vi "mainVI.vi"() -> ()   [LabVIEW 2019]
uses:
  controls/#typedef_StateMachine_States.ctl
  <vilib>/sound2/lvsound2.llb/Sampling Mode.ctl
  controls/#typedef_Waveform_Type.ctl
  <vilib>/sound2/lvsound2.llb/Sound Data Format.ctl
  <vilib>/sound2/lvsound2.llb/Sound Output Task ID.ctl
  controls/#typedef_Data_Cluster.ctl
  <vilib>/Utility/file.llb/Read Delimited Spreadsheet (string).vi
  <vilib>/sound2/lvsound2.llb/Sound Output Write (DBL Single).vi
panel:
  out "Main Data Cluster":T1={"Notes Frequency Array"=[], "Main Waveform Type"=enum."Sine", "Waveform"={"t0"=timestamp(0 s since 1904-01-01), "dt"=1.0, "Y"=[]}, "Main Current Note"=0, "Octave Range Offset"=0, "sound format"={"sample rate (S/s)"=22050.0, "number of channels"=2, "bits per sample"=16}, "Task ID"=0, "Note Duration"=0.0, "Volume"=0.0, "ADSR Envelope Cluster"={"Decay"=0, "Sustain"=0, "Attack"=0, "Release"=0}, "Playing?"=FALSE, "Pitch LFO"={"Rate"=0.0, "Ammount"=0.0}, "device ID"=0, "Filter Section"={"Lowpass Freq"=0.0, "Highpass Freq"=0.0, "Enable"=FALSE}, "Distortion"={"Distortion level"=0.0, "Enable"=FALSE}, "Secondary Waveform Type"=enum."Sine", "Secondary Frequency"=0.0, "Secondary Blend"=0.0, "Envelope XY Graph"={[], []}, "Buffer Number"=0, "End of Sequence?"=FALSE} {"task ID" format="%.0x"}
  out "error out":errorcluster
  out "ADSR Graph":cluster{dbl[], dbl[]}(graph)
  in  "Load Button":bool
  in  "Save Button":bool
  in  "Filter frequency":dbl(slide)=5.783132530120482 min=-0.0 max=1125.0 scale=1.0..1125.0 scale format="%#_5g"
  out "Waveform Graph":waveform(dbl)(graph)
  in  "Octave Range":u32(knob)=2 min=1 max=4 step=1 scale=1.0..4.0
  in  "Sub Volume":dbl(knob) scale=0.0..1.0
  in  "Sub Waveform Selection":u32(knob) max=4 step=1 scale=0.0..4.0
  in  "Sub Note Dial":dbl(knob) min=0.0 step=1.0 scale=0.0..12.0
  in  "Distortion level":dbl(slide) scale=0.0..100.0
  out "Distortion Enable LED":bool
  in  "Distortion Enable":bool
  out "Filter Enable LED":bool
  in  "Filter Enable":bool
  in  "Waveform Selection":u32(knob) max=4 step=1 scale=0.0..4.0
  in  "Pause Button":bool
  in  "Play Button":bool
  in  "Stop Button":bool
  in  "Volume":dbl(knob) scale=0.0..1.0
  in  "Sustain":i32(slide)=100 scale=10.0..100.0
  in  "Decay":i32(slide)=10 scale=10.0..100.0
  out "FFT Graph":cluster{"f0":dbl, "df":dbl, "magnitude":dbl[]}(graph)
  in  "Attack":i32(slide)=10 scale=10.0..100.0
  in  "Release":i32(slide)=10 scale=10.0..100.0
  in  "Settings Button":bool
  in  "Sequence legnth":dbl(knob)=10.0 scale=10.0..100.0
  in  "Dial 12":dbl(knob) scale=0.0..12.0
  in  "Dial 16":dbl(knob) scale=0.0..12.0
  in  "Dial 15":dbl(knob) scale=0.0..12.0
  in  "Dial 14":dbl(knob) scale=0.0..12.0
  in  "Dial 11":dbl(knob) scale=0.0..12.0
  in  "Dial 13":dbl(knob) scale=0.0..12.0
  in  "Dial 10":dbl(knob) scale=0.0..12.0
  in  "Dial 9":dbl(knob) scale=0.0..12.0
  in  "Dial 8":dbl(knob) scale=0.0..12.0
  in  "Dial 7":dbl(knob) scale=0.0..12.0
  in  "Dial 6":dbl(knob) scale=0.0..12.0
  in  "Dial 5":dbl(knob) scale=0.0..12.0
  in  "Dial 4":dbl(knob) scale=0.0..12.0
  in  "Dial 3":dbl(knob) scale=0.0..12.0
  in  "Dial 2":dbl(knob) scale=0.0..12.0
  in  "Dial 1":dbl(knob) min=1.0 step=1.0 scale=0.0..12.0
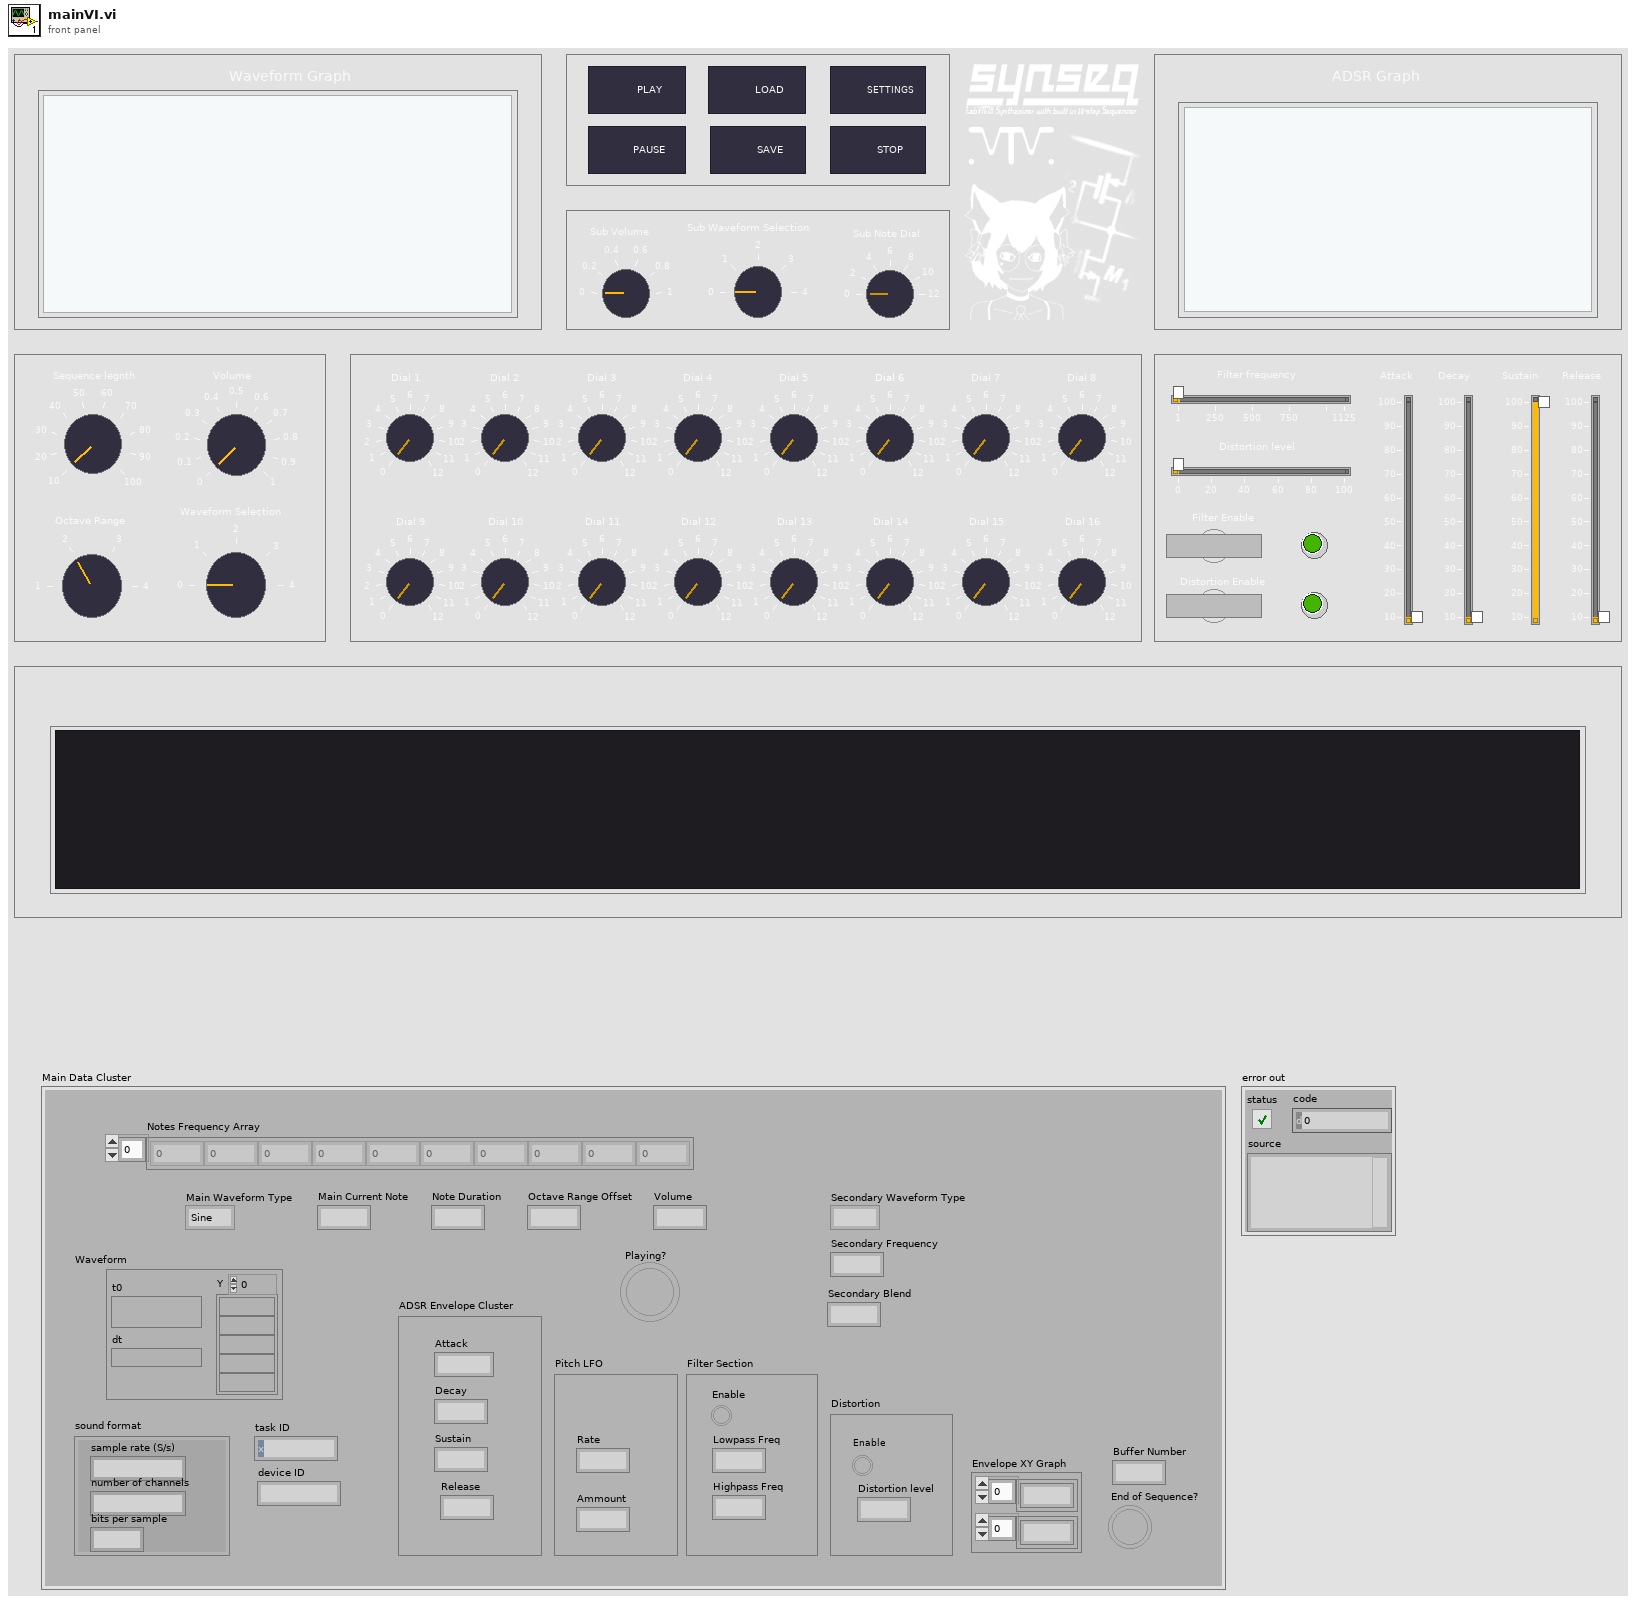
[diagram p1: front panel]
types:
  T1 = typedef "#typedef_Data_Cluster.ctl" = cluster{"Notes Frequency Array":dbl[], "Main Waveform Type":T2, "Waveform":waveform(dbl), "Main Current Note":i32, "Octave Range Offset":u32, "sound format":T3, "Task ID":T4, "Note Duration":dbl, "Volume":dbl, "ADSR Envelope Cluster":cluster{"Decay":i32, "Sustain":i32, "Attack":i32, "Release":i32}, "Playing?":bool, "Pitch LFO":cluster{"Rate":dbl, "Ammount":dbl}, "device ID":u32, "Filter Section":cluster{"Lowpass Freq":dbl, "Highpass Freq":dbl, "Enable":bool}, "Distortion":cluster{"Distortion level":dbl, "Enable":bool}, "Secondary Waveform Type":T2, "Secondary Frequency":dbl, "Secondary Blend":dbl, "Envelope XY Graph":cluster{dbl[], dbl[]}, "Buffer Number":i32, "End of Sequence?":bool}
  T2 = typedef "#typedef_Waveform_Type.ctl" = enum16{"Sine", "Saw", "Square", "Triangle", "Noise"}
  T3 = typedef "Sound Data Format.ctl" = cluster{"sample rate (S/s)":dbl, "number of channels":i32, "bits per sample":i32}
  T4 = typedef "Sound Output Task ID.ctl" = u32
  T5 = typedef "#typedef_StateMachine_States.ctl" = enum16{"Stop", "Idle", "Init", "Settings", "Write Data", "Read Data", "Play Data", "Err", "Load Sequence", "Save Sequence"}
  T6 = cluster{"Decay":i32, "Sustain":i32, "Attack":i32, "Release":i32}
  T7 = enum16{"open", "replace", "create", "open or create", "replace or create", "replace or create with confirmation"}
  T8 = typedef "Sampling Mode.ctl" = i32
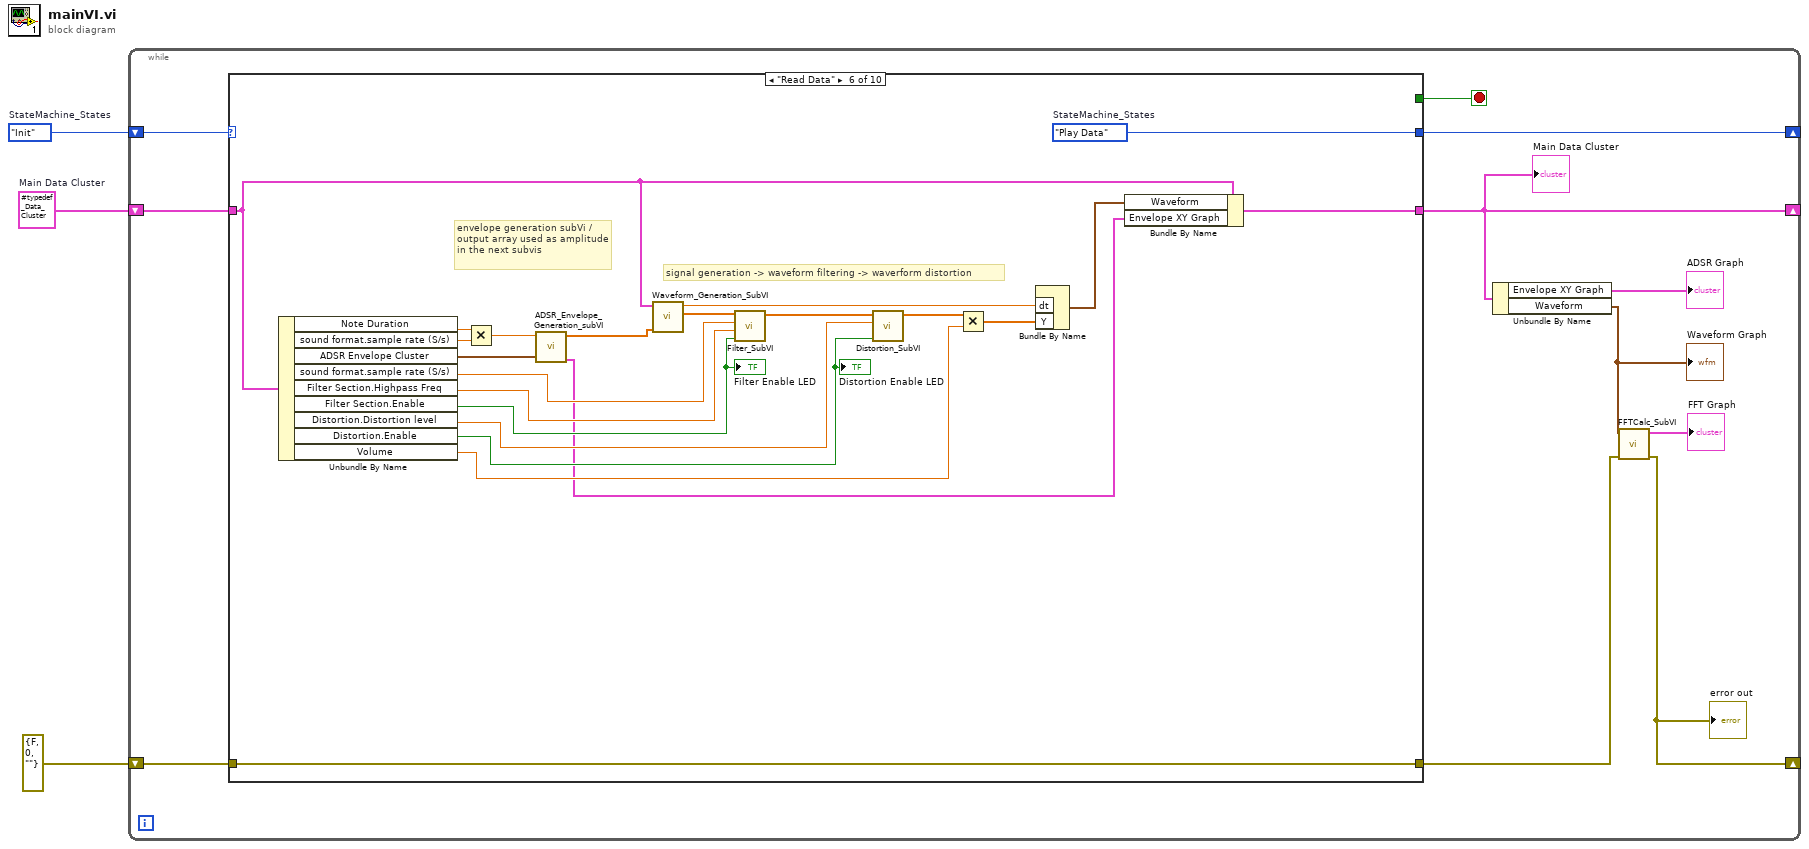
[diagram p0: block diagram]
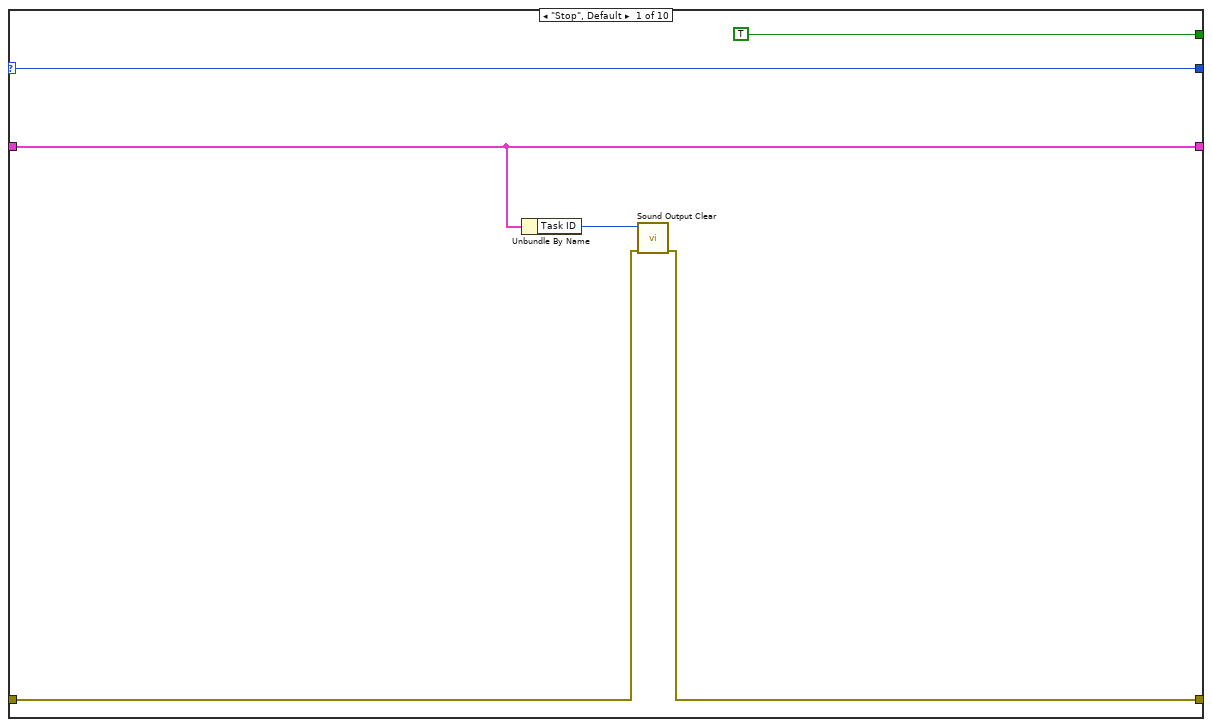
[diagram p2: hidden frame]
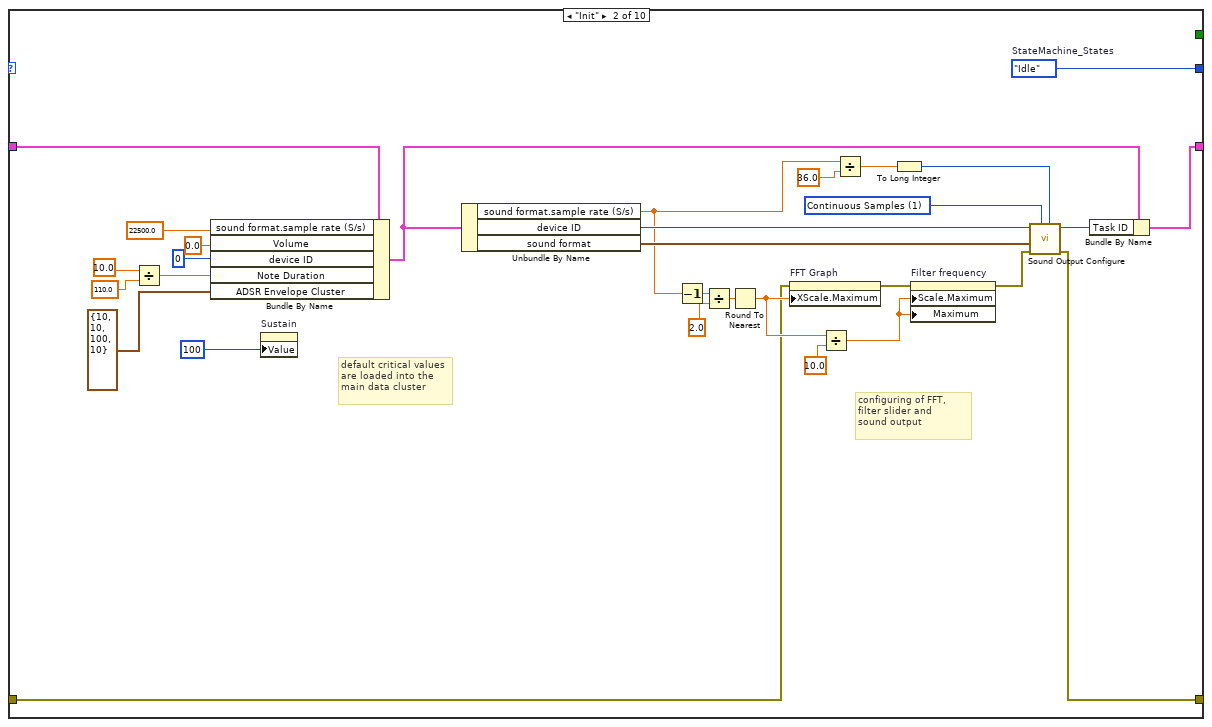
[diagram p3: hidden frame]
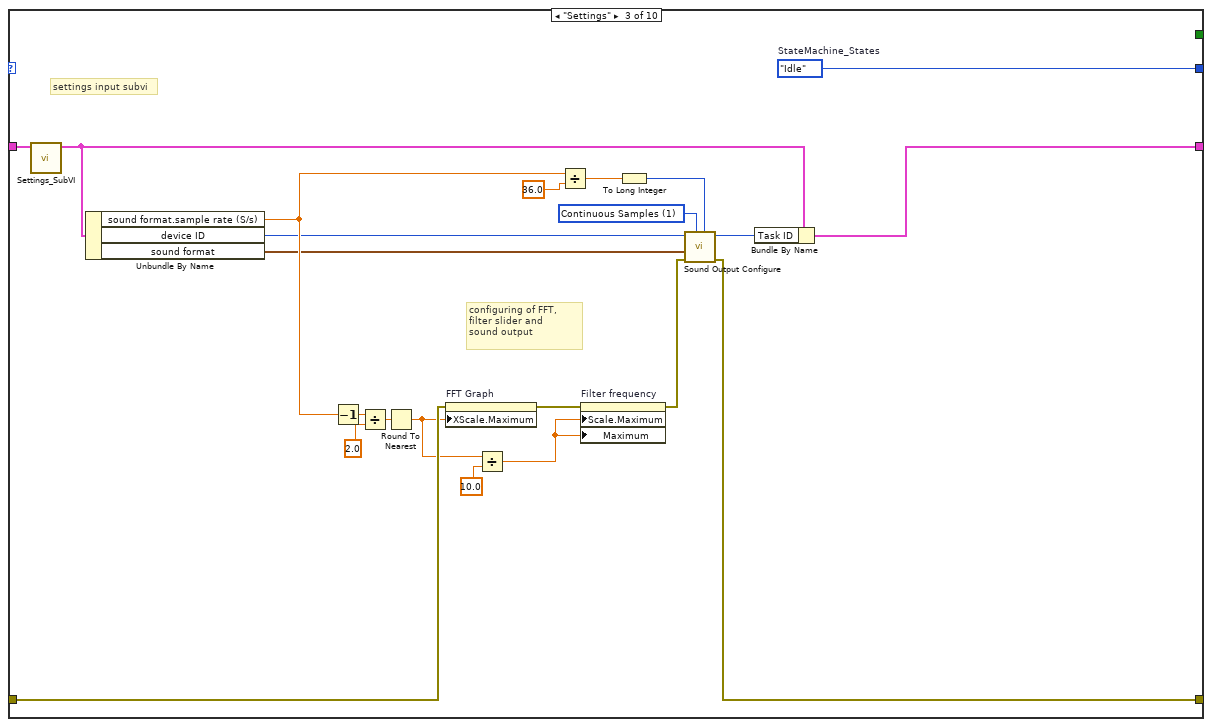
[diagram p4: hidden frame]
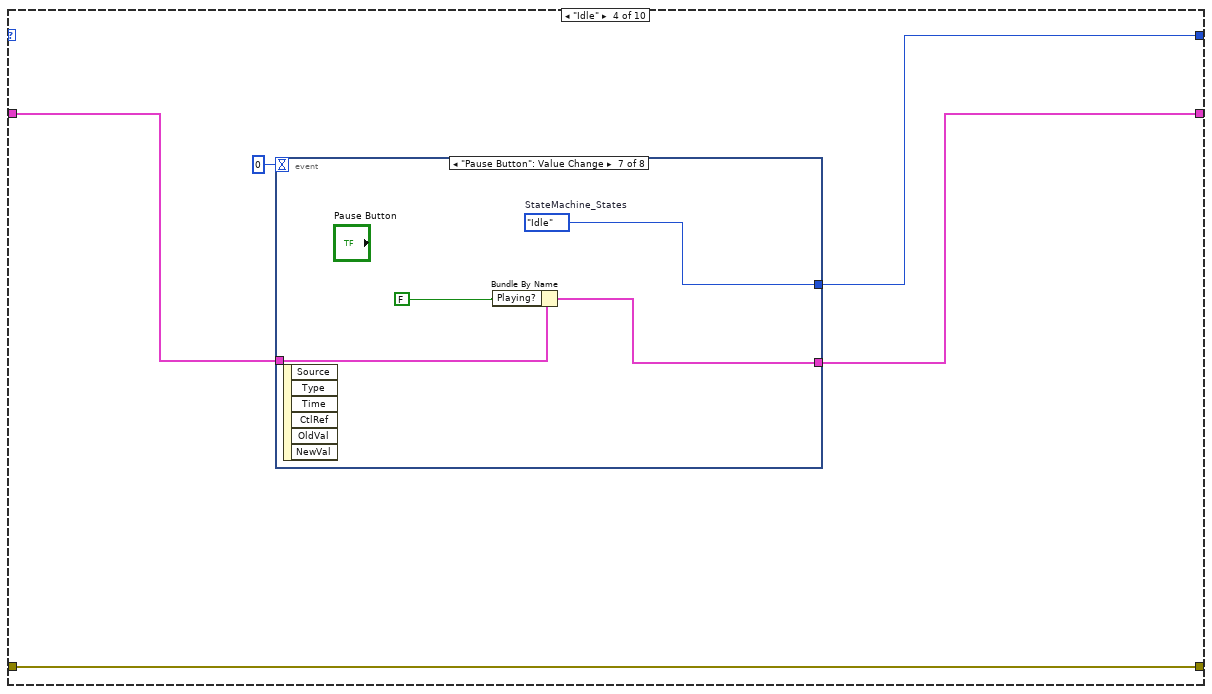
[diagram p5: hidden frame]
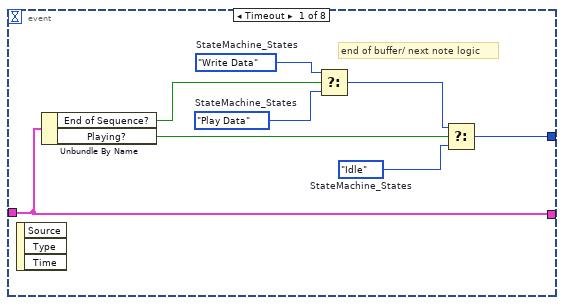
[diagram p6: hidden frame]
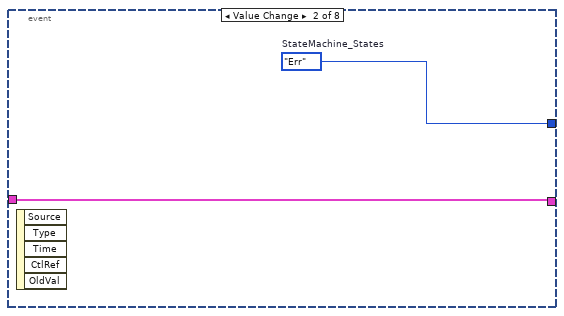
[diagram p7: hidden frame]
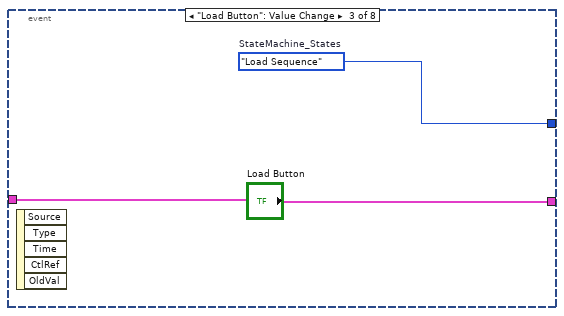
[diagram p8: hidden frame]
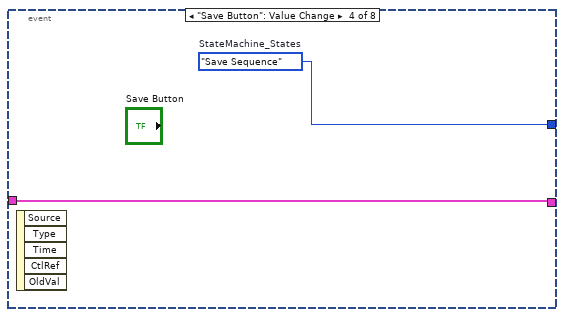
[diagram p9: hidden frame]
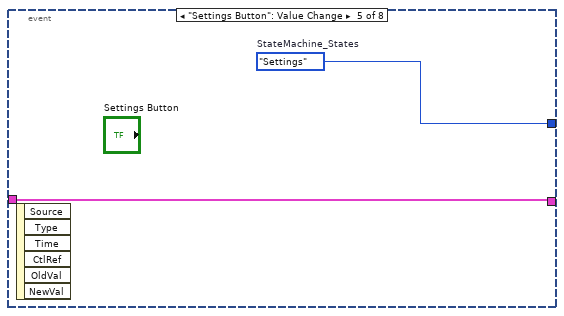
[diagram p10: hidden frame]
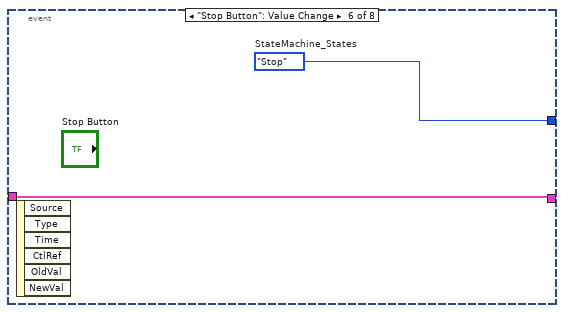
[diagram p11: hidden frame]
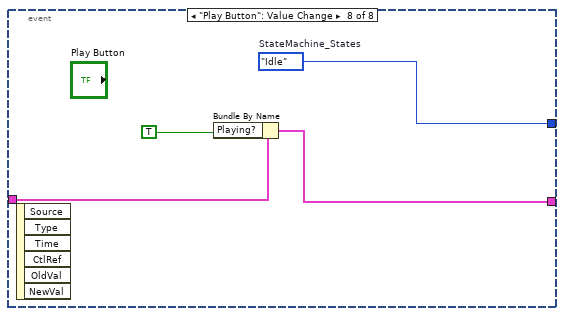
[diagram p12: hidden frame]
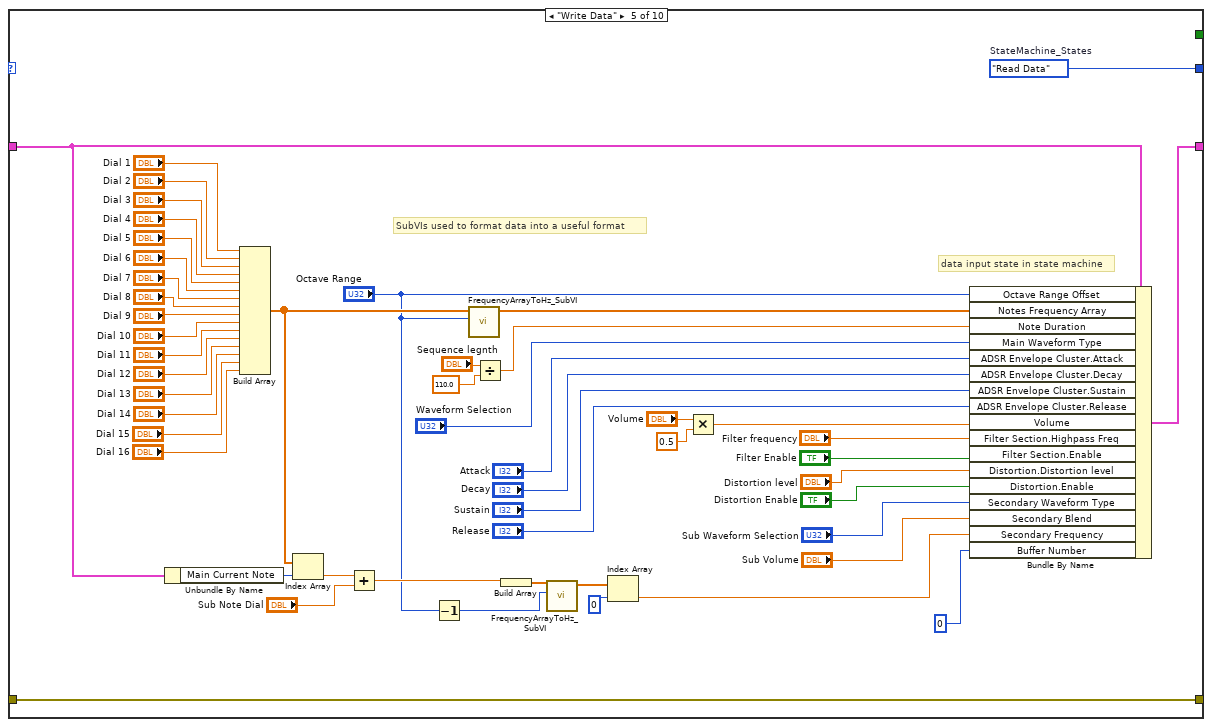
[diagram p13: hidden frame]
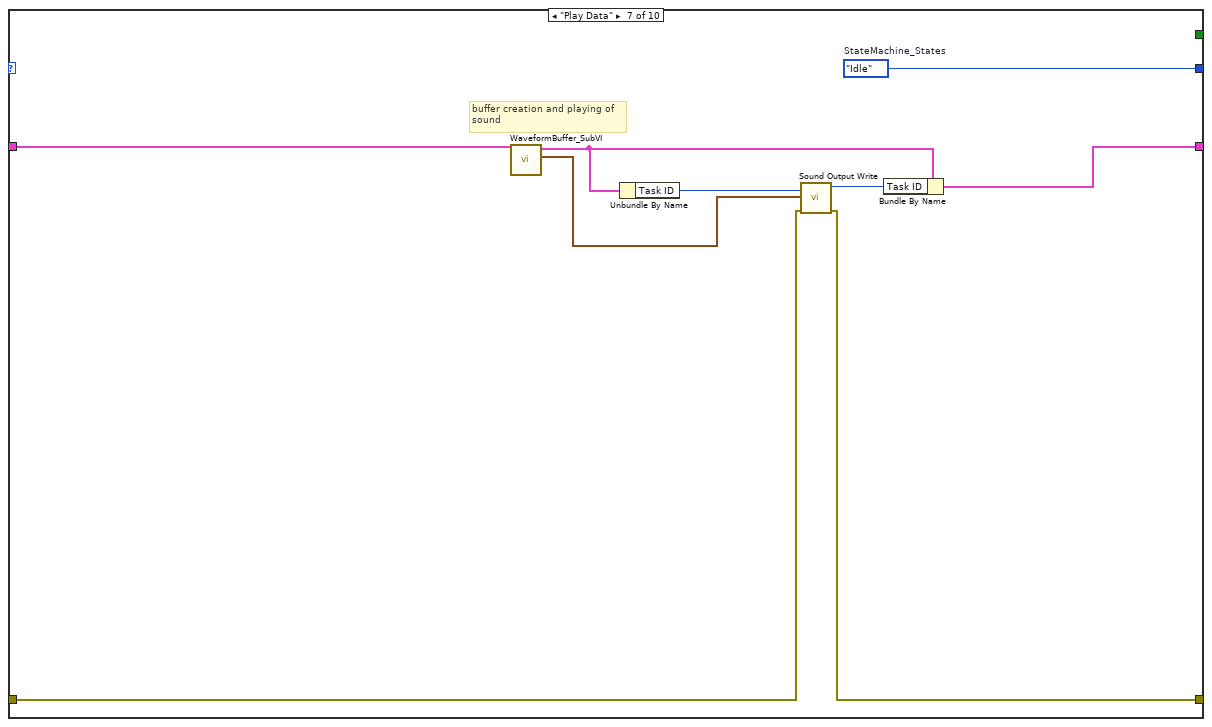
[diagram p14: hidden frame]
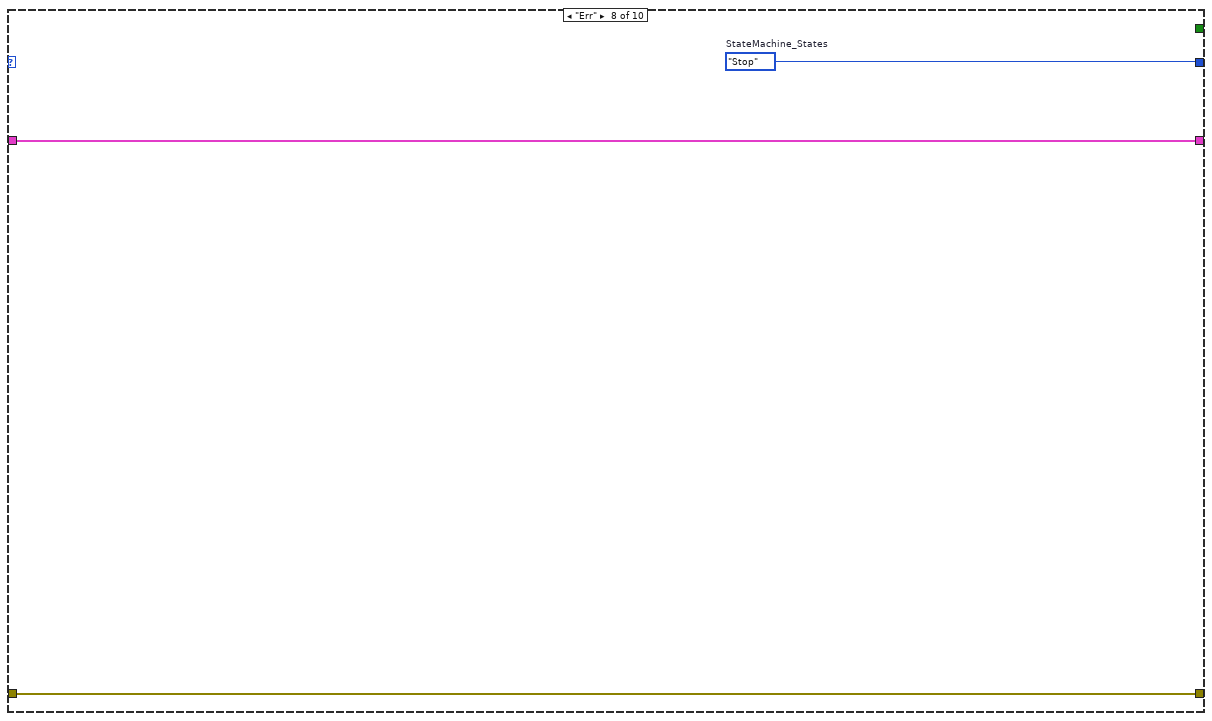
[diagram p15: hidden frame]
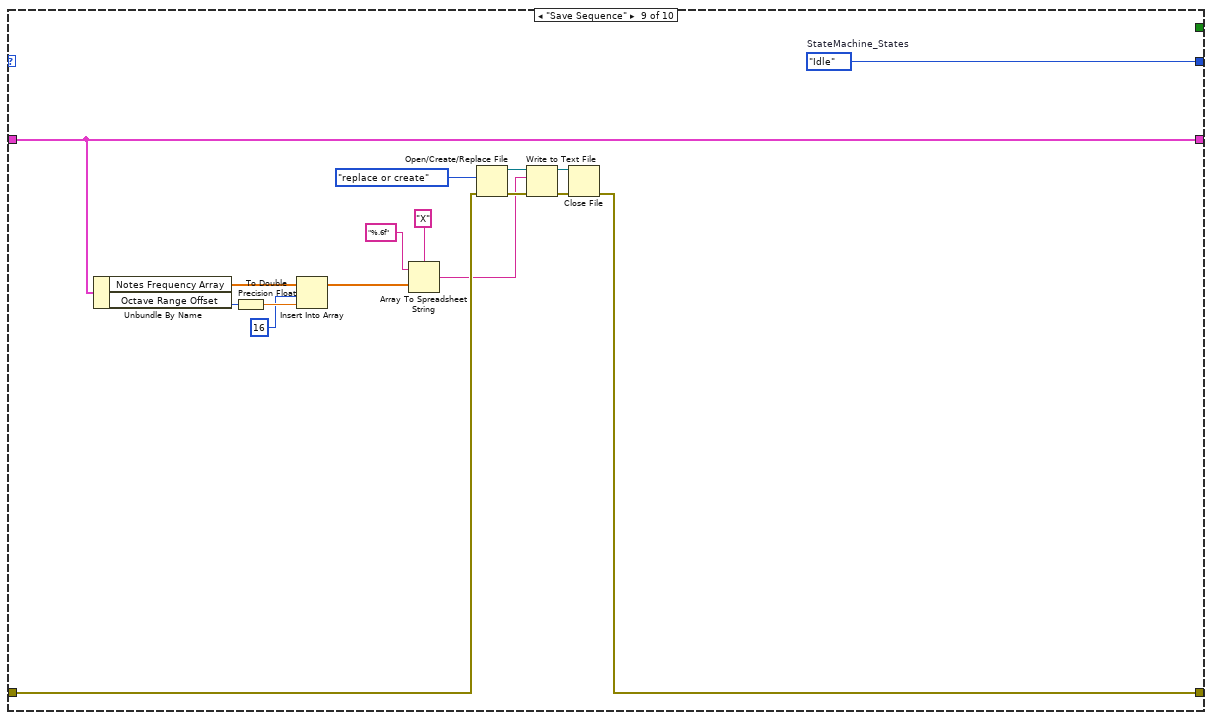
[diagram p16: hidden frame]
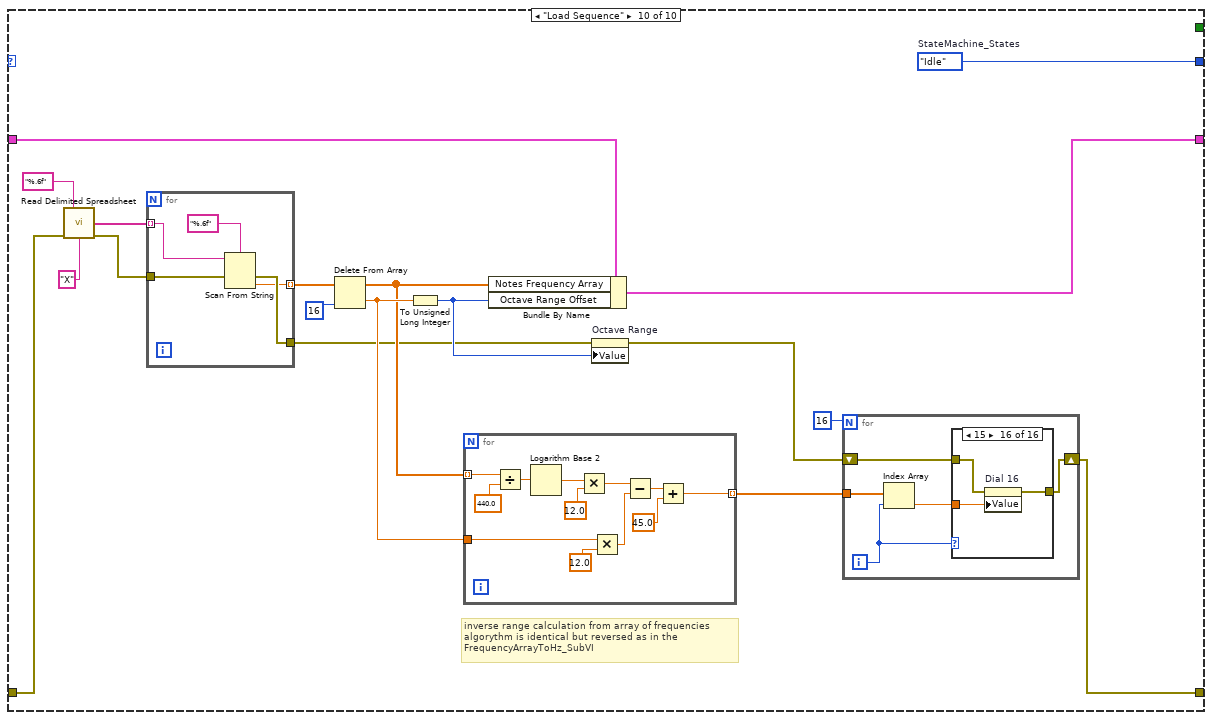
[diagram p17: hidden frame]
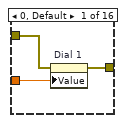
[diagram p18: hidden frame]
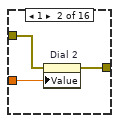
[diagram p19: hidden frame]
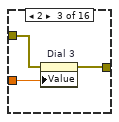
[diagram p20: hidden frame]
diagram:
  w2 = T1 {"Notes Frequency Array"=[], "Main Waveform Type"=enum."Sine", "Waveform"={"t0"=timestamp(0 s since 1904-01-01), "dt"=1.0, "Y"=[]}, "Main Current Note"=0, "Octave Range Offset"=0, "sound format"={"sample rate (S/s)"=22050.0, "number of channels"=2, "bits per sample"=16}, "Task ID"=0, "Note Duration"=0.0, "Volume"=0.0, "ADSR Envelope Cluster"={"Decay"=0, "Sustain"=0, "Attack"=0, "Release"=0}, "Playing?"=FALSE, "Pitch LFO"={"Rate"=0.0, "Ammount"=0.0}, "device ID"=0, "Filter Section"={"Lowpass Freq"=0.0, "Highpass Freq"=0.0, "Enable"=FALSE}, "Distortion"={"Distortion level"=0.0, "Enable"=FALSE}, "Secondary Waveform Type"=enum."Sine", "Secondary Frequency"=0.0, "Secondary Blend"=0.0, "Envelope XY Graph"={[], []}, "Buffer Number"=0, "End of Sequence?"=FALSE}  # Main Data Cluster
  w3 = #typedef_StateMachine_States."Init"  # StateMachine_States
  n1 = while {
    shift-right: [w11] -> _
    shift-left: w3 -> [w14]
    shift-right: [w9] -> _
    shift-left: w2 -> [w12]
    shift-right: [w5] -> _
    shift-left: errorcluster {"status"=FALSE, "code"=0, "source"=""} ("error out") -> [w10]
    stop <- w13 stop-if-true
    n2 = case shown="\"Read Data\"" w14 {
      selector: w14 -> [w19 _ _ _ _ _ _ _ _ _]
      tunnel: [w19 w50 w72 w77 w138 w154 w184 w185 w199 w222] -> w11
      tunnel: [TRUE _ _ _ _ _ _ _ _ _] -> w13
      tunnel: w12 -> [w18 w40 w71 w76 w108 w159 w178 w186 w194 w214]
      tunnel: [w18 w43 w51 w75 w107 w175 w183 w186 w194 w213] -> w9
      tunnel: w10 -> [w17 w30 w66 w73 w106 w157 w182 w187 w198 w220]
      tunnel: [w16 w41 w53 w73 w106 w157 w180 w187 w197 w206] -> w8
      frame "Stop", Default {
        n3 = Unbundle By Name(w18) -> ("Task ID"=w15:T4)
        n4 = call <vilib>:"Sound Output Clear.vi"("error in (no error)"=w17, "task ID"=w15) -> ("error out"=w16:errorcluster)  [unwired: 9 in]
      }
      frame "Init" {
        w49 = T8 1 items=["Finite Samples", "Continuous Samples"] ("sample mode")
        w50 = #typedef_StateMachine_States."Idle"  # StateMachine_States
        # "configuring of FFT, filter slider and\nsound output"
        # "default critical values are loaded into the main data cluster"
        n5 = Divide(x=10.0, y=110.0) -> (x/y=w24:dbl)
        n6 = Bundle By Name(cluster=w40, "sound format.sample rate (S/s)"=22500.0, "Volume"=0.0, "device ID"=u32 0, "Note Duration"=w24, "ADSR Envelope Cluster"=T6 {"Decay"=10, "Sustain"=10, "Attack"=100, "Release"=10}) -> (w39:T1)
        n7 = property on="Sustain" class="Slide (strict)"("Value"=100 ("Sustain")) -> ()  [unwired: 2 in, 2 out]
        n8 = Unbundle By Name(w39) -> ("sound format.sample rate (S/s)"=w29:dbl, "device ID"=w42:u32, "sound format"=w48:T3)
        n9 = Decrement(x=w29) -> (x-1=w35:dbl)
        n10 = Divide(x=w35, y=2.0) -> (x/y=w36:dbl)
        n11 = Round To Nearest(number=w36) -> (nearest integer value=w33:dbl)
        n12 = property on="FFT Graph" class="WFGraph (strict)"(error in=w30, "XScale.Maximum"=w33) -> (error out=w28:errorcluster)  [unwired: 1 in, 1 out]
        n13 = Divide(x=w33, y=10.0) -> (x/y=w32:dbl)
        n14 = Divide(x=w29, y=36.0) -> (x/y=w47:dbl)
        n15 = To Long Integer(number=w47) -> (32bit integer=w45:i32)
        n16 = property on="Filter frequency" class="Slide (strict)"(error in=w28, "Scale.Maximum"=w32, "Maximum"=w32) -> (error out=w31:errorcluster)  [unwired: 1 in, 1 out]
        n17 = call <vilib>:"Sound Output Configure.vi"("number of samples/ch"=w45, "sample mode"=w49, "error in (no error)"=w31, "sound format"=w48, "device ID"=w42) -> ("error out"=w41:errorcluster, "task ID"=w44:T4)  [unwired: 5 in]
        n18 = Bundle By Name(cluster=w39, "Task ID"=w44) -> (w43:T1)
      }
      frame "Settings" {
        w62 = T8 1 items=["Finite Samples", "Continuous Samples"] ("sample mode")
        w72 = #typedef_StateMachine_States."Idle"  # StateMachine_States
        # "settings input subvi"
        # "configuring of FFT, filter slider and\nsound output"
        n19 = call "Settings_SubVI.vi"("Main Data Cluster in"=w71) -> ("Main Data Cluster out"=w52:T1)  [unwired: 10 in]
        n20 = Unbundle By Name(w52) -> ("sound format.sample rate (S/s)"=w57:dbl, "device ID"=w56:u32, "sound format"=w55:T3)
        n21 = Decrement(x=w57) -> (x-1=w68:dbl)
        n22 = Divide(x=w68, y=2.0) -> (x/y=w69:dbl)
        n23 = Round To Nearest(number=w69) -> (nearest integer value=w65:dbl)
        n24 = property on="FFT Graph" class="WFGraph (strict)"(error in=w66, "XScale.Maximum"=w65) -> (error out=w64:errorcluster)  [unwired: 1 in, 1 out]
        n25 = Divide(x=w65, y=10.0) -> (x/y=w63:dbl)
        n26 = Divide(x=w57, y=36.0) -> (x/y=w61:dbl)
        n27 = property on="Filter frequency" class="Slide (strict)"(error in=w64, "Scale.Maximum"=w63, "Maximum"=w63) -> (error out=w54:errorcluster)  [unwired: 1 in, 1 out]
        n28 = To Long Integer(number=w61) -> (32bit integer=w59:i32)
        n29 = call <vilib>:"Sound Output Configure.vi"("number of samples/ch"=w59, "sample mode"=w62, "error in (no error)"=w54, "sound format"=w55, "device ID"=w56) -> ("error out"=w53:errorcluster, "task ID"=w58:T4)  [unwired: 5 in]
        n30 = Bundle By Name(cluster=w52, "Task ID"=w58) -> (w51:T1)
      }
      frame "Idle" {
        n31 = event shown="[6] \"Pause Button\": Value Change" {
          selector: _ -> [_ _ _ _ _ _ _ _]
          dyn-events: _ -> [_ _ _ _ _ _ _ _]
          timeout: 0 -> [_ _ _ _ _ _ _ _]
          tunnel: [w82 w86 w88 w90 w93 w94 w96 w100] -> w77
          tunnel: w76 -> [w85 w87 w89 w91 w92 w95 w99 w103]
          tunnel: [w85 w87 w89 w91 w92 w95 w98 w102] -> w75
          event Timeout {
            w78 = #typedef_StateMachine_States."Write Data"  # StateMachine_States
            w84 = #typedef_StateMachine_States."Idle"  # StateMachine_States
            w79 = #typedef_StateMachine_States."Play Data"  # StateMachine_States
            # "end of buffer/ next note logic"
            n32 = event-data() -> ()  [unwired: 1 in, 3 out]
            n33 = Unbundle By Name(w85) -> ("End of Sequence?"=w80:bool, "Playing?"=w83:bool)
            n34 = Select(t=w78, s=w80, f=w79) -> (s? t:f=w81:T5)
            n35 = Select(t=w81, s=w83, f=w84) -> (s? t:f=w82:T5)
          }
          event "error out.status": Value Change {
            w86 = #typedef_StateMachine_States."Err"  # StateMachine_States
            n36 = event-data() -> ()  [unwired: 1 in, 5 out]
          }
          event "Load Button": Value Change {
            w88 = #typedef_StateMachine_States."Load Sequence"  # StateMachine_States
            n37 = event-data() -> ()  [unwired: 1 in, 5 out]
          }
          event "Save Button": Value Change {
            w90 = #typedef_StateMachine_States."Save Sequence"  # StateMachine_States
            n38 = event-data() -> ()  [unwired: 1 in, 5 out]
          }
          event "Settings Button": Value Change {
            w93 = #typedef_StateMachine_States."Settings"  # StateMachine_States
            n39 = event-data() -> ()  [unwired: 1 in, 6 out]
          }
          event "Stop Button": Value Change {
            w94 = #typedef_StateMachine_States."Stop"  # StateMachine_States
            n40 = event-data() -> ()  [unwired: 1 in, 6 out]
          }
          event "Pause Button": Value Change {
            w96 = #typedef_StateMachine_States."Idle"  # StateMachine_States
            n41 = event-data() -> ()  [unwired: 1 in, 6 out]
            n42 = Bundle By Name(cluster=w99, "Playing?"=FALSE) -> (w98:T1)
          }
          event "Play Button": Value Change {
            w100 = #typedef_StateMachine_States."Idle"  # StateMachine_States
            n43 = event-data() -> ()  [unwired: 1 in, 6 out]
            n44 = Bundle By Name(cluster=w103, "Playing?"=TRUE) -> (w102:T1)
          }
        }
      }
      frame "Write Data" {
        w138 = #typedef_StateMachine_States."Read Data"  # StateMachine_States
        # "SubVIs used to format data into a useful format"
        # "data input state in state machine"
        n45 = Unbundle By Name(w108) -> ("Main Current Note"=w119:i32)
        n46 = Build Array("Dial 1", "Dial 2", "Dial 3", "Dial 4", "Dial 5", "Dial 6", "Dial 7", "Dial 8", "Dial 9", "Dial 10", "Dial 11", "Dial 12", "Dial 13", "Dial 14", "Dial 15", "Dial 16") -> (w116:dbl[])
        n47 = Index Array(array=w116, index=w119) -> (element=w114:dbl)
        n48 = Add(x=w114, y="Sub Note Dial") -> (x+y=w112:dbl)
        n49 = Decrement(x="Octave Range") -> (x-1=w111:u32)
        n50 = call "FrequencyArrayToHz_SubVI.vi"("Octave Range in"="Octave Range", "Notes array in"=w116) -> ("Frequency array out"=w132:dbl[])  [unwired: 9 in]
        n51 = Divide(x="Sequence legnth", y=110.0) -> (x/y=w128:dbl)
        n52 = Build Array(w112) -> (w115:dbl[])
        n53 = call "FrequencyArrayToHz_SubVI.vi"("Octave Range in"=w111, "Notes array in"=w115) -> ("Frequency array out"=w122:dbl[])  [unwired: 9 in]
        n54 = Index Array(array=w122, index=0) -> (element=w117:dbl)
        n55 = Multiply(x="Volume", y=0.5) -> (x*y=w130:dbl)
        n56 = Bundle By Name(cluster=w108, "Octave Range Offset"="Octave Range", "Notes Frequency Array"=w132, "Note Duration"=w128, "Main Waveform Type"="Waveform Selection", "ADSR Envelope Cluster.Attack"="Attack", "ADSR Envelope Cluster.Decay"="Decay", "ADSR Envelope Cluster.Sustain"="Sustain", "ADSR Envelope Cluster.Release"="Release", "Volume"=w130, "Filter Section.Highpass Freq"="Filter frequency", "Filter Section.Enable"="Filter Enable", "Distortion.Distortion level"="Distortion level", "Distortion.Enable"="Distortion Enable", "Secondary Waveform Type"="Sub Waveform Selection", "Secondary Blend"="Sub Volume", "Secondary Frequency"=w117, "Buffer Number"=0) -> (w107:T1)
      }
      frame "Read Data" {
        w154 = #typedef_StateMachine_States."Play Data"  # StateMachine_States
        # "envelope generation subVi / output array used as amplitude in the next subvis"
        # "signal generation -> waveform filtering -> waverform distortion"
        n57 = Unbundle By Name(w159) -> ("Note Duration"=w172:dbl, "sound format.sample rate (S/s)"=w173:dbl, "ADSR Envelope Cluster"=w171:T6, "sound format.sample rate (S/s)"=w170:dbl, "Filter Section.Highpass Freq"=w169:dbl, "Filter Section.Enable"=w168:bool, "Distortion.Distortion level"=w166:dbl, "Distortion.Enable"=w165:bool, "Volume"=w160:dbl)
        "Filter Enable LED" <- w168
        "Distortion Enable LED" <- w165
        n58 = Multiply(x=w172, y=w173) -> (x*y=w174:dbl)
        n59 = call "ADSR_Envelope_Generation_subVI.vi"("ADSR Envelope Cluster in"=w171, "Number of Samples in"=w174) -> ("Envelope XY Graph out"=w155:cluster{dbl[], dbl[]}, "Envelope Array out"=w158:dbl[])  [unwired: 8 in]
        n60 = call "Waveform_Generation_SubVI.vi"("ADSR in"=w158, "Main Data Cluster in"=w159) -> ("Signal Array out"=w163:dbl[], "dt out"=w164:dbl)  [unwired: 8 in]
        n61 = call "Filter_SubVI.vi"("Enable"=w168, "Highpass Freq"=w169, "sample rate (S/s)"=w170, "Signal Array"=w163) -> ("Filtered X"=w167:dbl[])  [unwired: 7 in]
        n62 = call "Distortion_SubVI.vi"("Enable"=w165, "Distortion level"=w166, "Signal"=w167) -> ("Distorted Signal"=w162:dbl[])  [unwired: 8 in]
        n63 = Multiply(x=w162, y=w160) -> (x*y=w161:dbl[])
        n64 = Bundle By Name("dt"=w164, "Y"=w161) -> (w156:waveform(dbl))  [unwired: 1 in]
        n65 = Bundle By Name(cluster=w159, "Waveform"=w156, "Envelope XY Graph"=w155) -> (w175:T1)
      }
      frame "Play Data" {
        w184 = #typedef_StateMachine_States."Idle"  # StateMachine_States
        # "buffer creation and playing of sound"
        n66 = call "WaveformBuffer_SubVI.vi"("Main Data Cluster in"=w178) -> ("waveform out"=w177:waveform(dbl), "Main Data Cluster out"=w176:T1)  [unwired: 9 in]
        n67 = Unbundle By Name(w176) -> ("Task ID"=w181:T4)
        n68 = call-poly <vilib>:"Sound Output Write.vi"("error in (no error)"=w182, "data"=w177, "task ID"=w181) -> ("error out"=w180:errorcluster, "task ID out"=w179:T4)  [unwired: 7 in]
        n69 = Bundle By Name(cluster=w176, "Task ID"=w179) -> (w183:T1)
      }
      frame "Err" {
        w185 = #typedef_StateMachine_States."Stop"  # StateMachine_States
      }
      frame "Save Sequence" {
        w199 = #typedef_StateMachine_States."Idle"  # StateMachine_States
        n70 = Unbundle By Name(w194) -> ("Notes Frequency Array"=w192:dbl[], "Octave Range Offset"=w189:u32)
        n71 = To Double Precision Float(number=w189) -> (double precision float=w191:dbl)
        n72 = Insert Into Array(array=w192, index=16, new element=w191) -> (w188:dbl[])
        n73 = Array To Spreadsheet String(delimiter (Tab)="X", array=w188, 3:"%.6f" ("format string")) -> (spreadsheet string=w193:string)
        n74 = Open/Create/Replace File(error in=w198, operation (0:open)=T7."replace or create") -> (refnum out=w201:refnum<file>, error out=w204:errorcluster)  [unwired: 4 in, 1 out]
        n75 = Write to Text File(file (use dialog)=w201, text=w193, error in=w204) -> (refnum out=w202:refnum<file>, error out=w203:errorcluster)  [unwired: 1 in, 1 out]
        n76 = Close File(refnum=w202, error in=w203) -> (error out=w197:errorcluster)  [unwired: 1 out]
      }
      frame "Load Sequence" {
        w222 = #typedef_StateMachine_States."Idle"  # StateMachine_States
        # "inverse range calculation from array of frequencies\nalgorythm is identical but reversed as in the FrequencyArrayToHz_SubVI"
        n77 = call-poly <vilib>:"Read Delimited Spreadsheet.vi"("format (%s)"="%.6f" ("format (%.3f)"), "error in (no error)"=w220, "delimiter (\\t)"="X" ("delimiter (\\t)")) -> ("first row"=w218:string[], "error out"=w217:errorcluster)  [unwired: 7 in, 4 out]
        n78 = for {
          tunnel: w218 -> [w292] mode=indexing
          tunnel: w217 -> [w290]
          tunnel: [w289] -> w207
          tunnel: [w288] -> w215 mode=indexing
          n79 = Scan From String(format string="%.6f", input string=w292, error in=w290) -> (error out=w289:errorcluster, output 1=w288:dbl)  [unwired: 2 in, 2 out]
        }
        n80 = Delete From Array(array=w215, index=16) -> (deleted portion=w212:dbl, array with subset deleted=w211:dbl[])  [unwired: 1 in]
        n81 = To Unsigned Long Integer(number=w212) -> (unsigned 32bit integer=w209:u32)
        n82 = for {
          tunnel: w212 -> [w281]
          tunnel: w211 -> [w277] mode=indexing
          tunnel: [w276] -> w205 mode=indexing
          n83 = Divide(x=w277, y=440.0) -> (x/y=w286:dbl)
          n84 = Logarithm Base 2(1:w286) -> (0:w285:dbl)
          n85 = Multiply(x=w285, y=12.0) -> (x*y=w283:dbl)
          n86 = Multiply(x=w281, y=12.0) -> (x*y=w280:dbl)
          n87 = Subtract(x=w283, y=w280) -> (x-y=w279:dbl)
          n88 = Add(x=w279, y=45.0) -> (x+y=w276:dbl)
        }
        n89 = Bundle By Name(cluster=w214, "Notes Frequency Array"=w211, "Octave Range Offset"=w209) -> (w213:T1)
        n90 = property on="Octave Range" class="Knob (strict)"(error in=w207, "Value"=w209) -> (error out=w208:errorcluster)  [unwired: 1 in, 1 out]
        n91 = for {
          N: 16 -> [_]
          tunnel: w205 -> [w227]
          shift-right: [w223] -> w206
          shift-left: w208 -> [w224]
          i -> [w226]
          n92 = Index Array(array=w227, index=w226) -> (element=w225:dbl)
          n93 = case shown="15" w226 {
            tunnel: w225 -> [w230 w233 w236 w239 w242 w245 w248 w251 w254 w257 w260 w263 w266 w269 w272 w275]
            tunnel: w224 -> [w229 w232 w235 w238 w241 w244 w247 w250 w253 w256 w259 w262 w265 w268 w271 w274]
            tunnel: [w228 w231 w234 w237 w240 w243 w246 w249 w252 w255 w258 w261 w264 w267 w270 w273] -> w223
            frame 0, Default {
              n94 = property on="Dial 1" class="Knob (strict)"(error in=w229, "Value"=w230) -> (error out=w228:errorcluster)  [unwired: 1 in, 1 out]
            }
            frame 1 {
              n95 = property on="Dial 2" class="Knob (strict)"(error in=w232, "Value"=w233) -> (error out=w231:errorcluster)  [unwired: 1 in, 1 out]
            }
            frame 2 {
              n96 = property on="Dial 3" class="Knob (strict)"(error in=w235, "Value"=w236) -> (error out=w234:errorcluster)  [unwired: 1 in, 1 out]
            }
            frame 3 {
              n97 = property on="Dial 4" class="Knob (strict)"(error in=w238, "Value"=w239) -> (error out=w237:errorcluster)  [unwired: 1 in, 1 out]
            }
            frame 4 {
              n98 = property on="Dial 5" class="Knob (strict)"(error in=w241, "Value"=w242) -> (error out=w240:errorcluster)  [unwired: 1 in, 1 out]
            }
            frame 5 {
              n99 = property on="Dial 6" class="Knob (strict)"(error in=w244, "Value"=w245) -> (error out=w243:errorcluster)  [unwired: 1 in, 1 out]
            }
            frame 6 {
              n100 = property on="Dial 7" class="Knob (strict)"(error in=w247, "Value"=w248) -> (error out=w246:errorcluster)  [unwired: 1 in, 1 out]
            }
            frame 7 {
              n101 = property on="Dial 8" class="Knob (strict)"(error in=w250, "Value"=w251) -> (error out=w249:errorcluster)  [unwired: 1 in, 1 out]
            }
            frame 8 {
              n102 = property on="Dial 9" class="Knob (strict)"(error in=w253, "Value"=w254) -> (error out=w252:errorcluster)  [unwired: 1 in, 1 out]
            }
            frame 9 {
              n103 = property on="Dial 10" class="Knob (strict)"(error in=w256, "Value"=w257) -> (error out=w255:errorcluster)  [unwired: 1 in, 1 out]
            }
            frame 10 {
              n104 = property on="Dial 11" class="Knob (strict)"(error in=w259, "Value"=w260) -> (error out=w258:errorcluster)  [unwired: 1 in, 1 out]
            }
            frame 11 {
              n105 = property on="Dial 12" class="Knob (strict)"(error in=w262, "Value"=w263) -> (error out=w261:errorcluster)  [unwired: 1 in, 1 out]
            }
            frame 12 {
              n106 = property on="Dial 13" class="Knob (strict)"(error in=w265, "Value"=w266) -> (error out=w264:errorcluster)  [unwired: 1 in, 1 out]
            }
            frame 13 {
              n107 = property on="Dial 14" class="Knob (strict)"(error in=w268, "Value"=w269) -> (error out=w267:errorcluster)  [unwired: 1 in, 1 out]
            }
            frame 14 {
              n108 = property on="Dial 15" class="Knob (strict)"(error in=w271, "Value"=w272) -> (error out=w270:errorcluster)  [unwired: 1 in, 1 out]
            }
            frame 15 {
              n109 = property on="Dial 16" class="Knob (strict)"(error in=w274, "Value"=w275) -> (error out=w273:errorcluster)  [unwired: 1 in, 1 out]
            }
          }
        }
      }
    }
    "Main Data Cluster" <- w9
    n110 = Unbundle By Name(w9) -> ("Envelope XY Graph"=→"ADSR Graph":cluster{dbl[], dbl[]}, "Waveform"=w6:waveform(dbl))
    "Waveform Graph" <- w6
    n111 = call "FFTCalc_SubVI.vi"("error in (no error)"=w8, "Waveform"=w6) -> ("error out"=w5:errorcluster, "Power Spectrum / PSD"=→"FFT Graph":cluster{"f0":dbl, "df":dbl, "magnitude":dbl[]})  [unwired: 8 in]
    "error out" <- w5
  }
